vi "Draw Line Realtime 2D.vi"(6 "Voltage":dbl, 7 "Litho Point":cluster{dbl, dbl}, 8 "error in (no error)":errorcluster, 9 "ColorRamp in":refnum<vi>, 10 "Litho Point Old":cluster{dbl, dbl}, 11 "Refnum in":T1) -> (0 "error out":errorcluster, 3 "Refnum out":T1)   [LabVIEW 2020]
doc: "This VI draws a line on the 2D realtime IMAQ image."
uses:
  <vilib>/vision/Image Controls.llb/IMAQ Image.ctl
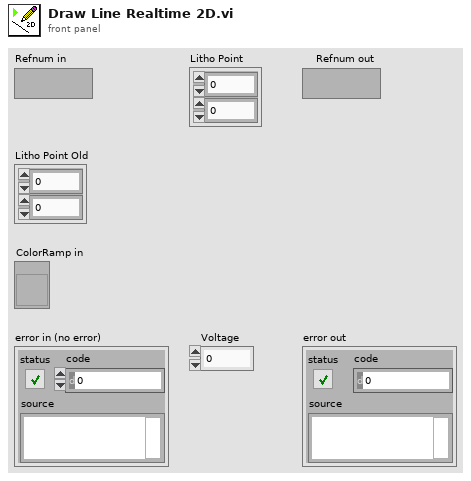
[diagram p1: front panel]
types:
  T1 = typedef "IMAQ Image.ctl" = refnum<image>
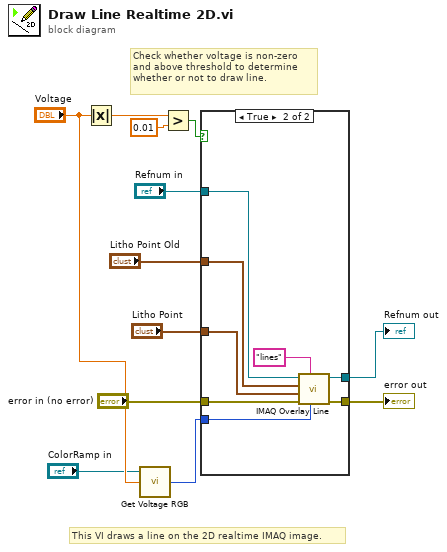
[diagram p0: block diagram]
diagram:
  # "This VI draws a line on the 2D realtime IMAQ image."
  # "Check whether voltage is non-zero\nand above threshold to determine\nwhether or not to draw line."
  n1 = Absolute Value(x="Voltage") -> (abs(x)=w2:dbl)
  n2 = call "Get Voltage RGB.vi"("Voltage"="Voltage", "ColorRamp in"="ColorRamp in") -> ("RGB Value"=w9:u32)  [unwired: 1 in, 2 out]
  n3 = Greater?(x=w2, y=0.01) -> (0:w11:bool)
  n4 = case shown="True" w11 {
    tunnel: "error in (no error)" -> [w14 w22]
    tunnel: "Refnum in" -> [w13 w21]
    tunnel: "Litho Point Old" -> [_ w19]
    tunnel: "Litho Point" -> [_ w18]
    tunnel: w9 -> [_ w17]
    tunnel: [w13 w16] -> w4
    tunnel: [w14 w15] -> w5
    frame False {
    }
    frame True {
      n5 = call "IMAQ Overlay Line"("Color"=w17, "Group"="lines", "error in (no error)"=w22, "End Point"=w18, "Start Point"=w19, "Image"=w21) -> ("error out"=w15:errorcluster, "Image Out"=w16:T1)  [unwired: 4 in]
    }
  }
  "error out" <- w5
  "Refnum out" <- w4
